vi "simx Get UI Event Button.vi"(6 "operationMode":i32, 7 "auxValues":i32, 8 "error in (no error)":errorcluster, 9 "uiEventButtonID":i32, 10 "uiHandle":i32, 11 "clientID":i32) -> (0 "error out":errorcluster, 1 "uiEventButtonID out":i32, 3 "function return":i32, 5 "auxValues out":i32)   [LabVIEW 2019, in "PXL_V-REP.lvlib"]
doc: "EXTAPI_DLLEXPORT simxInt simxGetUIEventButton(simxInt clientID,simxInt uiHandle,simxInt* uiEventButtonID,simxInt* auxValues,simxInt operationMode);"
uses:
  PXL_V-REP.lvlib
  <userlib>/V-REP/remoteApi.dll
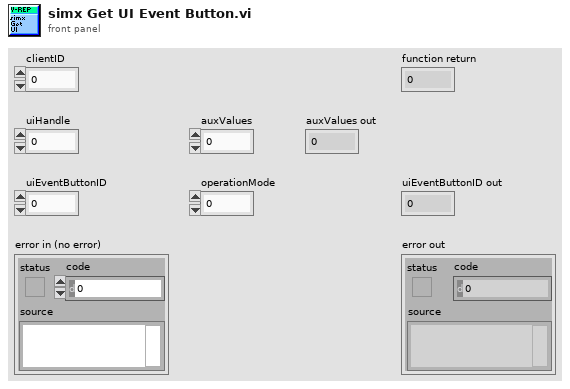
[diagram p1: front panel]
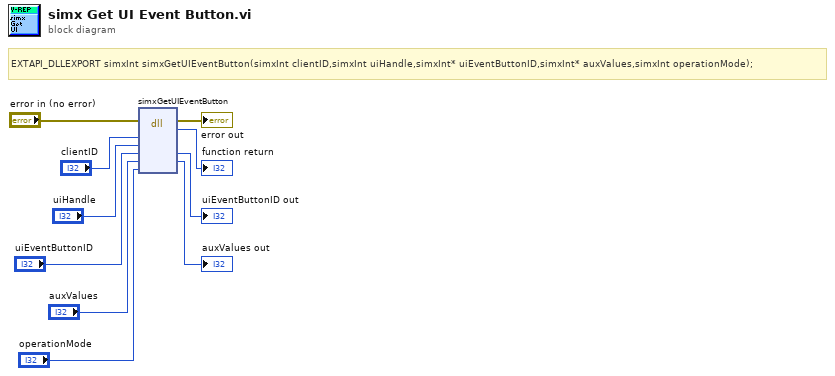
[diagram p0: block diagram]
diagram:
  # "EXTAPI_DLLEXPORT simxInt simxGetUIEventButton(simxInt clientID,simxInt uiHandle,simxInt* uiEventButtonID,simxInt* auxValues,simxInt operationMode);"
  n1 = dll-call lib="C:/Program Files (x86)/National Instruments/LabVIEW 2019/user.lib/V-REP/remoteApi.*" fn="simxGetUIEventButton"(error in="error in (no error)", "clientID"="clientID", "uiHandle"="uiHandle", "uiEventButtonID"="uiEventButtonID", "auxValues"="auxValues", "operationMode"="operationMode") -> (error out=→"error out":errorcluster, →"function return":i32, "uiEventButtonID"=→"uiEventButtonID out":i32, "auxValues"=→"auxValues out":i32)  [unwired: 5 in, 1 out]
